vi "Data Producer Worker Template_Start.vi"(0 "Data Producer Worker Template In":refnum<class "Data Producer Worker Template.lvclass">, 1 "Data Buffer Depth (-1: unlimited)":i32=-1, 5 "Instrument Address":string, 11 "error in":errorcluster) -> (4 "Data Producer Worker Template Out":refnum<class "Data Producer Worker Template.lvclass">, 15 "error out":errorcluster)   [LabVIEW 2013, in "Data Producer Worker Template.lvclass"]
uses:
  Data Producer Worker Template.lvclass
  Data Producer Worker Template_Data Queue.ctl
  Data Producer Worker Template.lvclass/Data Producer Worker Template.ctl
  Data Producer Worker Template_Worker.vi
panel:
  # "Inputs"
  # "Outputs"
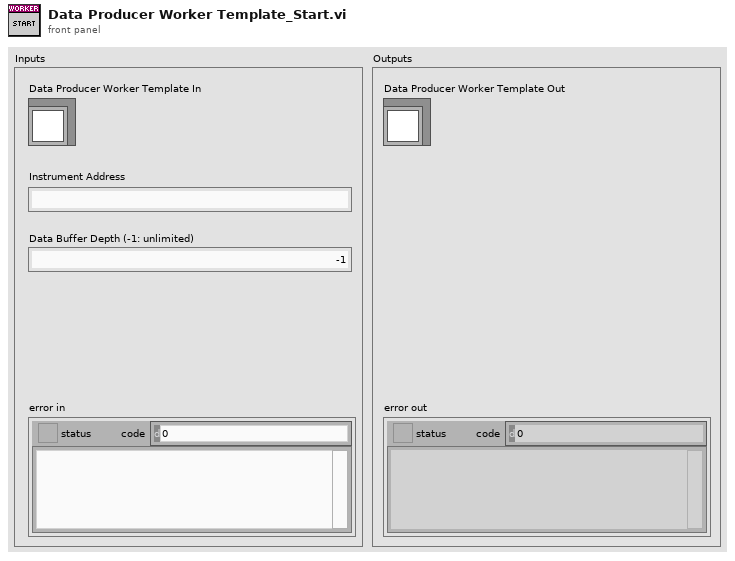
[diagram p1: front panel]
types:
  T1 = typedef "Data Producer Worker Template.lvclass/Data Producer Worker Template_Data Queue.ctl" = refnum<queue>
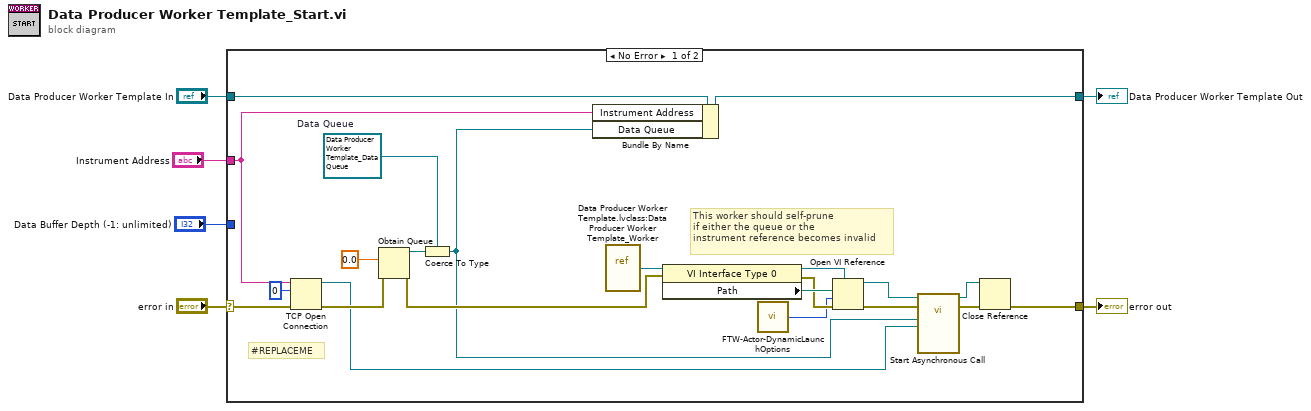
[diagram p0: block diagram]
diagram:
  n1 = case shown="No Error" "error in" {
    selector: "error in" -> [w18 w30]
    tunnel: [w15 w30] -> w6
    tunnel: "Data Producer Worker Template In" -> [w21 w29]
    tunnel: [w14 w29] -> w3
    tunnel: "Instrument Address" -> [w10 _]
    tunnel: "Data Buffer Depth (-1: unlimited)" -> [_ _]
    frame No Error {
      w13 = T1 refnum  # Data Queue
      # "#REPLACEME"
      # "This worker should self-prune\nif either the queue or the\ninstrument reference becomes invalid"
      n2 = TCP Open Connection(address=w10, remote port or service name=u16 0, error in (no error)=w18) -> (connection ID=w8:refnum<k5>, error out=w11:errorcluster)  [unwired: 2 in]
      n3 = Obtain Queue(element data type=0.0, error in (no error)=w11) -> (queue out=w19:refnum<queue>, error out=w20:errorcluster)  [unwired: 3 in, 1 out]
      n4 = Coerce To Type(0:w19, 1:w13) -> (2:w9:T1)
      n5 = Bundle By Name(cluster=w21, "Instrument Address"=w10, "Data Queue"=w9) -> (w14:refnum<class "Data Producer Worker Template.lvclass">)
      n6 = vi-ref "Data Producer Worker Template.lvclass:Data Producer Worker Template_Worker.vi"() -> (w28:refnum<vi>)
      n7 = property class="VI Interface Type 0"(reference=w28, error in=w20) -> (reference out=w27:refnum<vi>, error out=w24:errorcluster, "Path"=w26:path)
      n8 = call "FTW-Actor-DynamicLaunchOptions.vi"() -> ("Open VI Ref Options"=w23:i32)
      n9 = Open VI Reference(type specifier VI Refnum (for type only)=w27, vi path=w26, options=w23, error in (no error)=w24) -> (vi reference=w22:refnum<vi>, error out=w25:errorcluster)  [unwired: 2 in]
      n10 = call-by-ref "Start Asynchronous Call"(reference=w22, error in=w25, "Data Queue"=w9, "connection ID"=w8) -> (reference out=w17:refnum<vi>, error out=w16:errorcluster)  [unwired: 14 in]
      n11 = Close Reference(reference=w17, error in (no error)=w16) -> (error out=w15:errorcluster)
    }
    frame Error {
    }
  }
  "error out" <- w6
  "Data Producer Worker Template Out" <- w3
